vi "Joypad Loop.vi"() -> ()   [LabVIEW 2012]
doc: "This vi connects to a Joystick via Microsoft's Human Interface Devices and passes the necessary controls to the \"Remote\" variables \nSee Block Diagram:\n1. Quarry about available joystick\n2. Search for the joystick with the specified device\n3. If no match is found, then pass an error, then try and initialize the device\n4. Use a timed wile loop to save recourse, just looping and poling the joystick data is capable of high loop speeds\n5. Get Joystick sensor data\n6. Set the Trigger enable condition and pass along the XY data\n7. Normalize the values and use a running average to smooth out the control\n8. Apply expo weight for less sensitive control and zero out dead stick offset \n9. Set XY data\n10. XY plot is data binding to network variable for the XY plot on HUD from the Remote tab\n11. Use a stop button titled \"stop?\" so that the LabVIEW script can stop the vi\n12. Close the Joystick connection\n-Ruffin White\n-Kyle Green"
uses:
  <vilib>/Platform/TimedLoop/XDataNode/timing_clust.ctl
  <vilib>/Platform/TimedLoop/XDataNode/nitl_modes.ctl
  <vilib>/Platform/TimedLoop/XDataNode/wakeup.ctl
  <vilib>/Utility/inputDevices.llb/closeJoystick.vi
  <vilib>/Utility/inputDevices.llb/joystickAcquire.vi
  <vilib>/Platform/TimedLoop/XDataNode/XDataNode.xnode
  <vilib>/Platform/TimedLoop/XDataNode/XDNodeRunTimeDep.lvlib
panel:
  out "VI Name 2":string
  in  "Expo %":i32(slide)=1 scale=0.0..100.0
  out "X and Y":cluster{"X":dbl, "Y":dbl}
  out "Listed Devices":T1(array[cluster])
  out "Analog Stick":cluster{dbl, dbl}[](graph)
  out "error out":errorcluster
  in  "stop?":bool
  in  "Device Name":string="Controller (XBOX 360 For Windows)" caption="Give the exact \"divice name\" string of the joypad you would like to use."
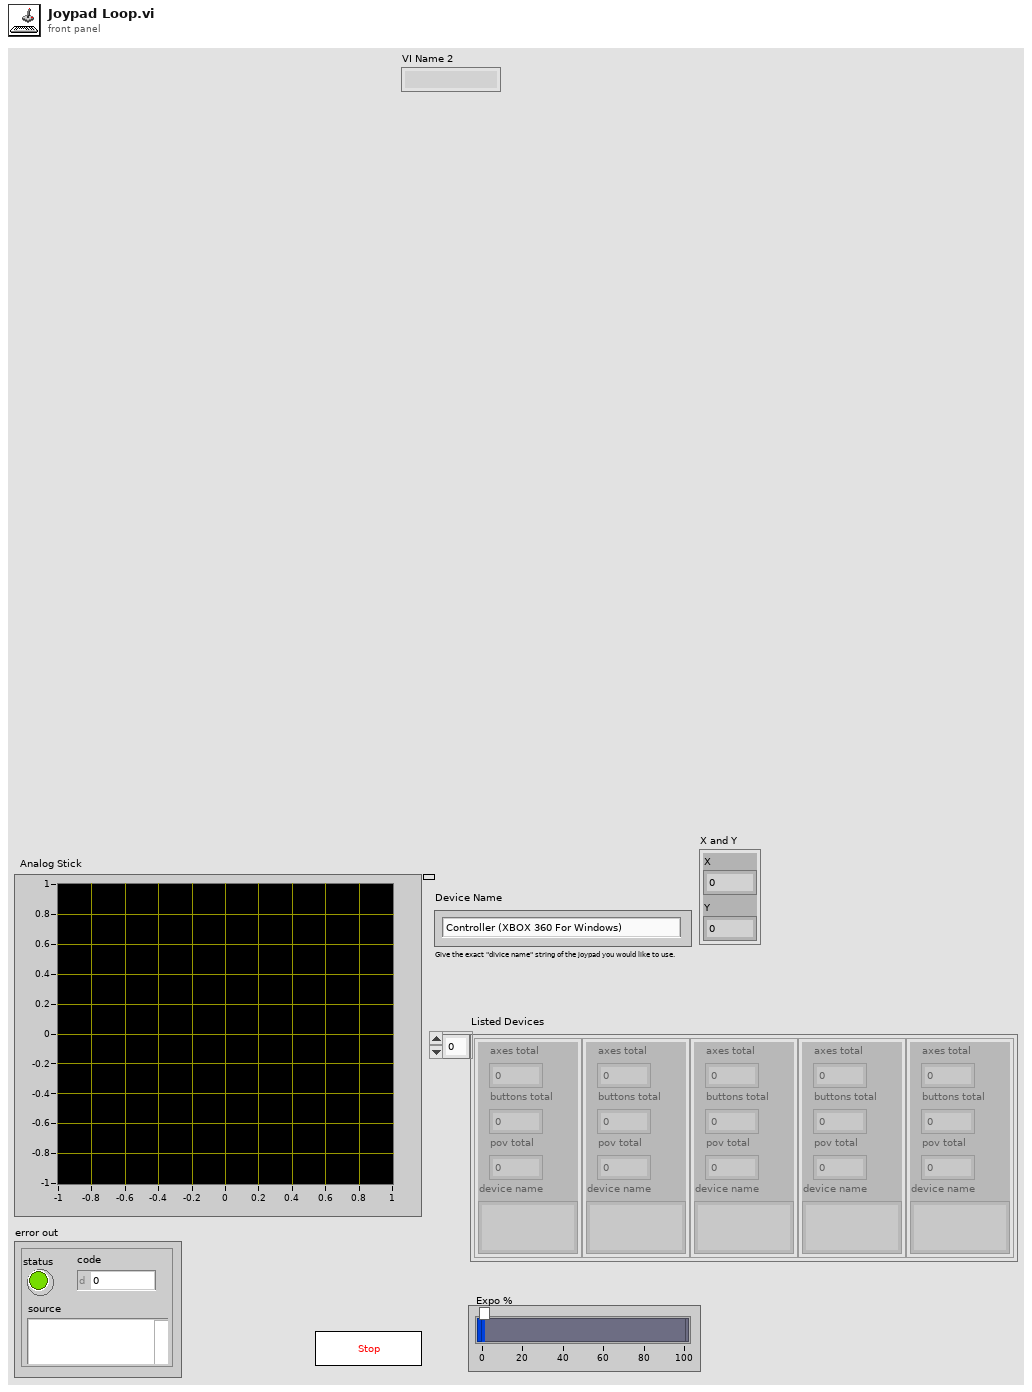
[diagram p1: front panel]
types:
  T1 = cluster{"axes total":u32, "buttons total":u32, "pov total":u32, "device name":string}[]
  T2 = typedef "XDNodeRunTimeDep.lvlib/timing_clust.ctl" = cluster{"Expected End [f-1]":u64, "Actual End [f-1]":u64, "Finished Late? [f-1]":bool, "Expected End [i-1]":u64, "Actual End [i-1]":u64, "Finished Late? [i-1]":bool, "Expected Start [i]":u64, "Actual Start [i]":u64, "Expected Start [f]":u64, "Actual Start [f]":u64, "Source Name":string, "Structure Name":string, "Period":i64, "Deadline":i64, "Offset":i64, "Start":i64, "Priority":i32, "Timeout":i32, "Mode":T3, "Wakeup Reason":T4, "Error":errorcluster, "Source Type":string, "Secondary Source Type":string, "Global End Time":u64, "Global Start Time":u64, "Frame Duration":u64, "Iteration Duration":u64, "Assigned CPU":i32, "I/O Scan Engine Mode":u32}
  T3 = typedef "XDNodeRunTimeDep.lvlib/nitl_modes.ctl" = enum32{"No Change", "Process missed periods, maintain original phase", "Discard missed periods, maintain original phase", "Process missed periods, ignore original phase", "Discard missed periods, ignore original phase"}
  T4 = typedef "XDNodeRunTimeDep.lvlib/wakeup.ctl" = enum32{"Normal", "Aborted", "Asynchronous wakeup", "Timing source error", "Timed loop error", "Timeout"}
  T5 = cluster{"X axis":i32, "Y axis":i32, "Z axis":i32, "X axis rotation":i32, "Y axis rotation":i32, "Z axis rotation":i32, "U axis":i32, "V axis":i32}
  T6 = cluster{"button 1":bool, "button 2":bool, "button 3":bool, "button 4":bool, "button 5":bool, "button 6":bool, "button 7":bool, "button 8":bool, "button 9":bool, "button 10":bool, "button 11":bool, "button 12":bool, "button 13":bool, "button 14":bool, "button 15":bool, "button 16":bool, "button 17":bool, "button 18":bool, "button 19":bool, "button 20":bool, "button 21":bool, "button 22":bool, "button 23":bool, "button 24":bool, "button 25":bool, "button 26":bool, "button 27":bool, "button 28":bool, "button 29":bool, "button 30":bool, "button 31":bool, "button 32":bool}
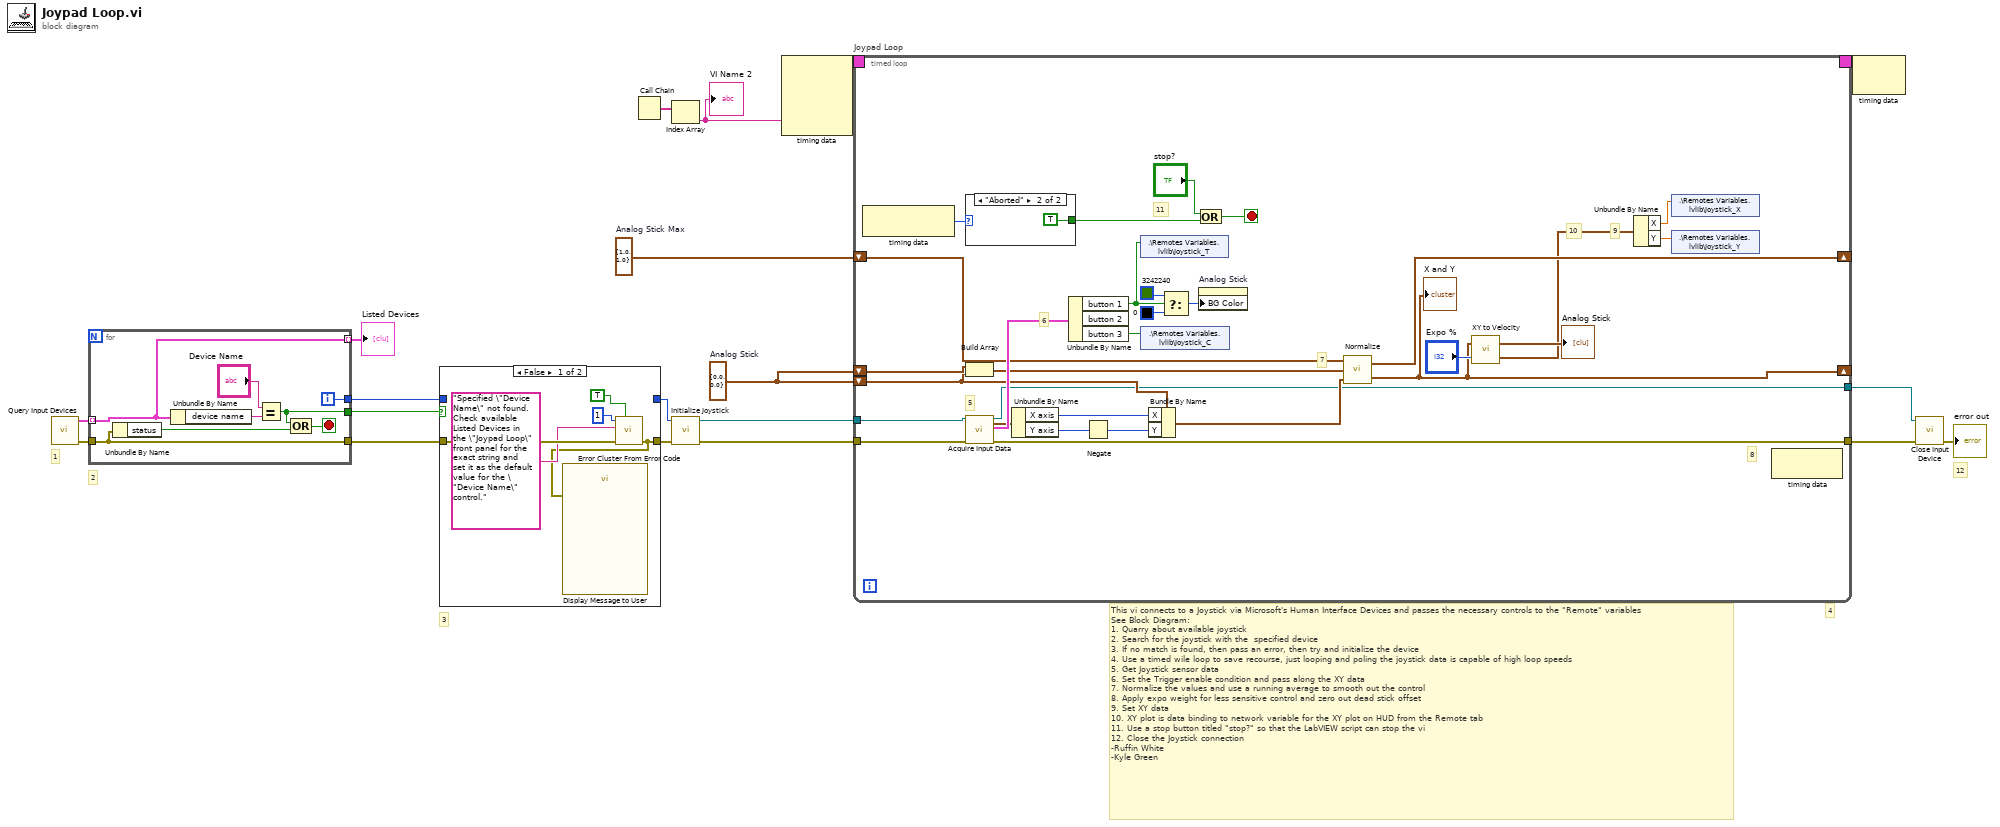
[diagram p0: block diagram]
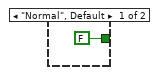
[diagram p2: hidden frame]
diagram:
  w6 = cluster{"X":dbl, "Y":dbl} {"X"=1.0, "Y"=1.0}  # Analog Stick Max
  w4 = cluster{"X":dbl, "Y":dbl} {"X"=0.0, "Y"=0.0}  # Analog Stick
  # "This vi connects to a Joystick via Microsoft's Human Interface Devices and passes the necessary controls to the \"Remote\" variables   \nSee Block Diagram:\n1.\tQuarry about available joystick\n2.\tSearch for the joystick with the  specified device\n3.\tIf no match is found, then pass an error, then try and initialize the device\n4.\tUse a timed wile loop to save recourse, just looping and poling the joystick data is capable of high loop speeds\n5.\tGet Joystick sensor data\n6.\tSet the Trigger enable condition and pass along the XY data\n7.\tNormalize the values and use a running average to smooth out the control\n8.\tApply expo weight for less sensitive control and zero out dead stick offset \n9.\tSet XY data\n10.\tXY plot is data binding to network variable for the XY plot on HUD from the Remote tab\n11.\tUse a stop button titled \"stop?\" so that the LabVIEW script can stop the vi\n12.\tClose the Joystick connection\n-Ruffin White\n-Kyle Green"
  # "12"
  # "4"
  # "3"
  # "2"
  # "1"
  n1 = call <vilib>:"Query Input Devices.vi"() -> ("error out"=w12:errorcluster, "joystick info"=w15:T1)  [unwired: 8 in, 2 out]
  n2 = for {
    tunnel: w15 -> [w20] mode=indexing
    tunnel: [w25] -> w14
    tunnel: [w22] -> w13
    tunnel: w12 -> [w23]
    tunnel: [w23] -> w11
    tunnel: [w20] -> w10 mode=indexing
    i -> [w25]
    stop <- w24 stop-if-true
    n3 = Unbundle By Name(w23) -> ("status"=w21:bool)
    n4 = Unbundle By Name(w20) -> ("device name"=w26:string)
    n5 = Equal?(x="Device Name", y=w26) -> (x = y?=w22:bool)
    n6 = Compound Arithmetic op=OR(w22, w21) -> (w24:bool)
  }
  "Listed Devices" <- w10
  n7 = case shown="False" w13 {
    tunnel: w14 -> [_ w34]
    tunnel: [_ w34] -> w9
    tunnel: w11 -> [w32 w33]
    tunnel: [w28 w33] -> w3
    frame False {
      n8 = call <vilib>:"Error Cluster From Error Code.vi"("show call chain? (False)"=TRUE, "error in (no error)"=w32, "error message (\"\")"="Specified \"Device Name\" not found. Check available Listed Devices in the \"Joypad Loop\" front panel for the exact string and set it as the default value for the \"Device Name\" control." ("error message (\"\")"), "error code (0)"=1) -> ("error out"=w28:errorcluster)  [unwired: 5 in]
      n9 = call "Display Message to User"("error in (no error)"=w28) -> ()  [unwired: 9 in, 2 out]
    }
    frame True {
    }
  }
  n10 = Call Chain() -> (call chain=w2:string[])
  n11 = Index Array(array=w2) -> (element=w1:string)  [unwired: 1 in]
  "VI Name 2" <- w1
  n12 = call <vilib>:"Initialize Joystick.vi"("error in (no error)"=w3, "device index"=w9) -> ("error out"=w16:errorcluster, "device ID"=w19:refnum<k1>)  [unwired: 8 in]
  n13 = node-c288(w1) -> (w8:T2)  [unwired: 3 in]
  n14 = timed-loop "Joypad Loop" {
    tunnel: w19 -> [w63]
    tunnel: [w58] -> w17
    tunnel: w16 -> [w61]
    shift-right: [w38] -> _
    shift-left: w4 -> [w55]
    timing: w8 -> [_]
    timing-out: [_] -> w7
    shift-right: [w42] -> _
    shift-left: w6 -> [w53]
    shift-left: w4 -> [w52]
    tunnel: [w50] -> w5
    stop <- w57 stop-if-true
    # "7"
    # "11"
    # "10"
    # "9"
    # "8"
    # "6"
    # "5"
    n15 = node-c288() -> (w36:T4)  [unwired: 1 in]
    n16 = case shown="\"Aborted\"" w36 {
      tunnel: [FALSE TRUE] -> w35
      frame "Normal", Default {
      }
      frame "Aborted" {
      }
    }
    n17 = Build Array(w55, w52) -> (w54:cluster{"X":dbl, "Y":dbl}[])
    n18 = call-poly <vilib>:"Acquire Input Data.vi"("device ID"=w63, "error in (no error)"=w61) -> ("device ID"=w50:refnum<k1>, "axis info"=w62:T5, "button info"=w64:T6, "error out"=w58:errorcluster)  [unwired: 13 in, 1 out]
    n19 = Unbundle By Name(w62) -> ("X axis"=w49:i32, "Y axis"=w45:i32)
    n20 = Unbundle By Name(w64) -> ("button 1"=w37:bool, "button 3"=w43:bool)  [unwired: 1 out]
    n21 = Negate(x=w45) -> (-x=w44:i32)
    n22 = shared-variable ".\\Remotes Variables.lvlib\\Joystick_T"(w37) -> ()  [unwired: 1 in, 1 out]
    n23 = shared-variable ".\\Remotes Variables.lvlib\\Joystick_C"(w43) -> ()  [unwired: 1 in, 1 out]
    n24 = Bundle By Name(cluster=w52, "X"=w49, "Y"=w44) -> (w51:cluster{"X":dbl, "Y":dbl})
    n25 = Select(t=u32 3242240, s=w37, f=u32 0) -> (s? t:f=w48:u32)
    n26 = property on="Analog Stick" class="XYGraph (strict)"("BG Color"=w48) -> ()  [unwired: 2 in, 2 out]
    n27 = Compound Arithmetic op=OR("stop?", w35) -> (w57:bool)
    n28 = call "Normalize.vi"("Analog Stick"=w51, "Past Analog Stick"=w54, "Analog Stick Max"=w53) -> ("Normalized Analog Stick Out"=w38:cluster{"X":dbl, "Y":dbl}, "Analog Stick Max Out"=w42:cluster{"X":dbl, "Y":dbl})
    "X and Y" <- w38
    n29 = call "XY to Velocity.vi"("Expo"="Expo %", "Nunchuk Analog Stick In"=w38) -> ("X and Y"=w39:cluster{"X":dbl, "Y":dbl}, "Nunchuk Analog Stick"=→"Analog Stick":cluster{dbl, dbl}[])
    n30 = Unbundle By Name(w39) -> ("X"=w60:dbl, "Y"=w59:dbl)
    n31 = shared-variable ".\\Remotes Variables.lvlib\\Joystick_X"(w60) -> ()  [unwired: 1 in, 1 out]
    n32 = shared-variable ".\\Remotes Variables.lvlib\\Joystick_Y"(w59) -> ()  [unwired: 1 in, 1 out]
    n33 = node-c288() -> ()  [unwired: 1 in, 1 out]
  }
  n34 = node-c288(w7) -> ()  [unwired: 1 out]
  n35 = call-poly <vilib>:"Close Input Device.vi"("error in (no error)"=w17, "device ID"=w5) -> ("error out"=→"error out":errorcluster)  [unwired: 8 in]
